vi "Chart-Map Graph Coords.vi"(8 "error in (no error)":errorcluster, 10 "XY":cluster{"X":dbl, "Y":dbl}, 11 "XY Graph Ref":refnum<vi>) -> (0 "error out":errorcluster, 2 "Coords":cluster{"X":i32, "Y":i32})   [LabVIEW 2020]
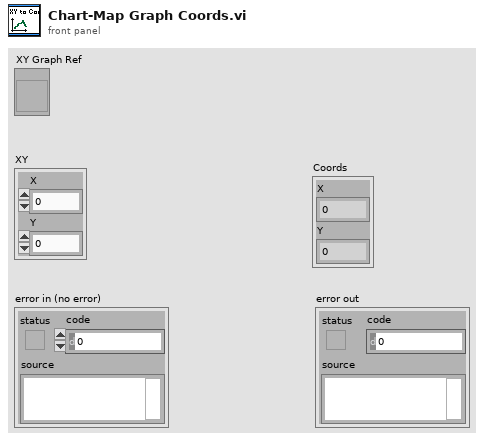
[diagram p1: front panel]
types:
  T1 = typedef "LVRectTypeDef.ctl" = cluster{"Left":i16, "Top":i16, "Right":i16, "Bottom":i16}
  T2 = typedef "LVPoint32TypeDef.ctl" = cluster{"Horizontal":i32, "Vertical":i32}
  T3 = cluster{"Left":i32, "Top":i32, "Right":i32, "Bottom":i32}
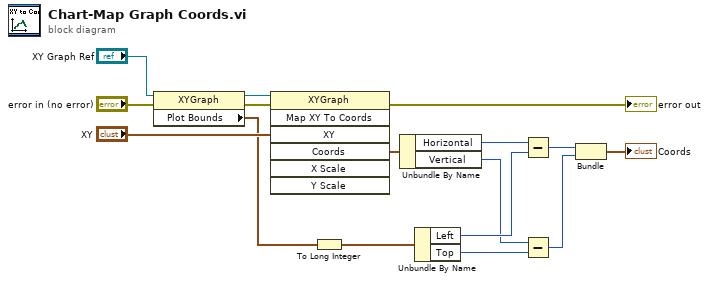
[diagram p0: block diagram]
diagram:
  n1 = property on="Property Node" class="XYGraph"(reference="XY Graph Ref", error in="error in (no error)") -> (reference out=w11:refnum<vi>, error out=w13:errorcluster, "Plot Bounds"=w8:T1)
  n2 = invoke on="Invoke Node" class="XYGraph" method="Map XY To Coords"(reference=w11, error in=w13, "XY"="XY") -> (error out=→"error out":errorcluster, "Coords"=w10:T2)  [unwired: 4 in, 5 out]
  n3 = To Long Integer(number=w8) -> (32bit integer=w7:T3)
  n4 = Unbundle By Name(w10) -> ("Horizontal"=w9:i32, "Vertical"=w5:i32)
  n5 = Unbundle By Name(w7) -> ("Left"=w6:i32, "Top"=w4:i32)
  n6 = Subtract(x=w9, y=w6) -> (x-y=w3:i32)
  n7 = Subtract(x=w5, y=w4) -> (x-y=w2:i32)
  n8 = Bundle(w3, w2) -> (→"Coords":cluster{i32, i32})  [unwired: 1 in]
